vi "Image_from_name.vi"(8 "error in (no error)":errorcluster, 10 "Chemical Name":string) -> (0 "error out":errorcluster, 1 "24-bit pixmap":u32[][](array[numeric]) format="%x", 2 "Downloaded Picture":picture)   [LabVIEW 2015]
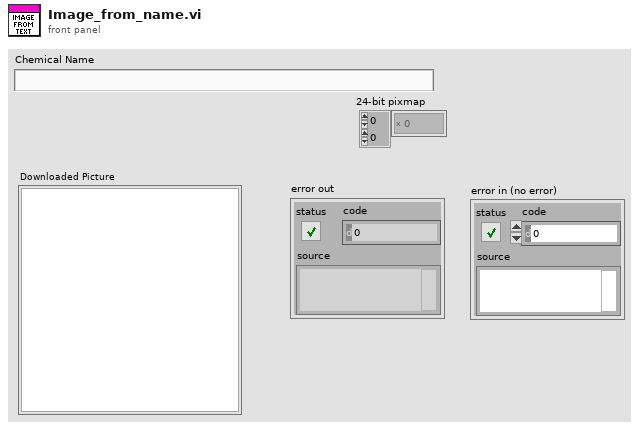
[diagram p1: front panel]
types:
  T1 = enum16{"open", "open or create", "create or replace", "create", "open (read only)"}
  T2 = typedef "imagedata.ctl" = cluster{"image type":i32, "image depth":i32, "image":u8[], "mask":u8[], "colors":u32[], "Rectangle":cluster{"left":i16, "top":i16, "right":i16, "bottom":i16}}
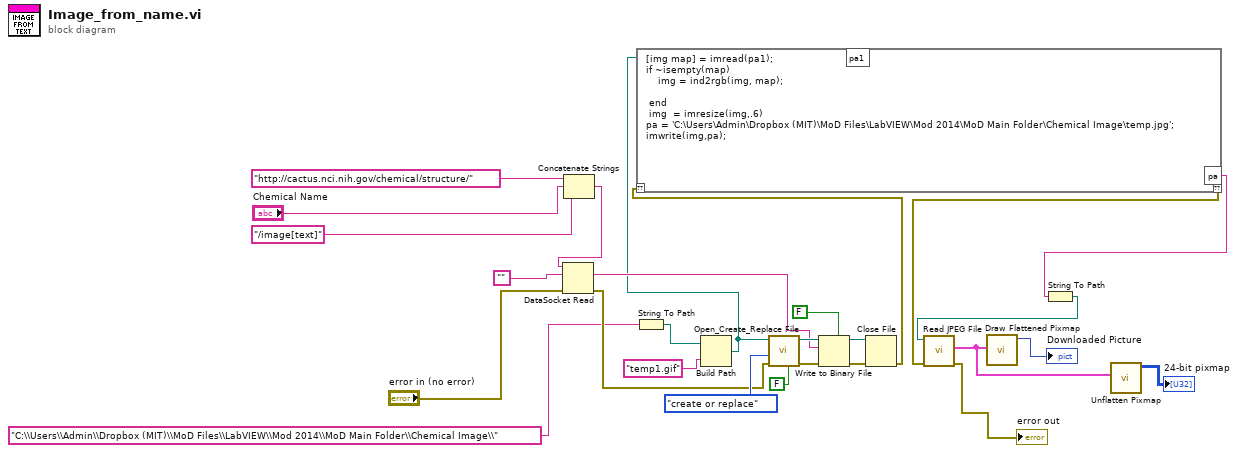
[diagram p0: block diagram]
diagram:
  n1 = Concatenate Strings("http://cactus.nci.nih.gov/chemical/structure/", "Chemical Name", "/image[text]") -> (w5:string)
  n2 = DataSocket Read(8:"error in (no error)", 10:"", 11:w5) -> (0:w18:errorcluster, 2:w14:string)  [unwired: 2 in, 5 out]
  n3 = String To Path(string="C:\\Users\\Admin\\Dropbox (MIT)\\MoD Files\\LabVIEW\\Mod 2014\\MoD Main Folder\\Chemical Image\\") -> (path=w1:path)
  n4 = Build Path(base path=w1, name or relative path="temp1.gif") -> (appended path=w9:path)
  n5 = call <vilib>:"Open_Create_Replace File.vi"("advisory dialog? (display:T)"=FALSE, "error in (no error)"=w18, "function (open:0)"=T1."create or replace", "file path"=w9) -> ("error out"=w24:errorcluster, "refnum"=w25:refnum<file>)  [unwired: 3 in, 3 out]
  n6 = Write to Binary File(file (use dialog)=w25, data=w14, error in=w24, 5:FALSE ("prepend array or string size? (T)")) -> (refnum out=w21:refnum<file>, error out=w20:errorcluster)  [unwired: 3 out]
  n7 = Close File(refnum=w21, error in=w20) -> (error out=w12:errorcluster)  [unwired: 1 out]
  n8 = script code="[img map] = imread(pa1);\nif ~isempty(map)\n    img = ind2rgb(img, map);\n   \n end\n img  = imresize(img,.6)\npa = 'C:\\Users\\Admin\\Dropbox (MIT)\\MoD Files\\LabVIEW\\Mod 2014\\MoD Main Folder\\Chemical Image\\temp.jpg';\nimwrite(img,pa);"("??"=w12, "pa1"=w9) -> ("??"=w11:errorcluster, "pa"=w13:string)
  n9 = String To Path(string=w13) -> (path=w10:path)
  n10 = call <vilib>:"Read JPEG File.vi"("error in (no error)"=w11, "path to JPEG file"=w10) -> ("error out"=→"error out":errorcluster, "image data"=w3:T2)  [unwired: 8 out]
  n11 = call <vilib>:"Draw Flattened Pixmap.vi"("image data"=w3) -> ("new picture"=→"Downloaded Picture":picture)  [unwired: 3 in, 5 out]
  n12 = call <vilib>:"Unflatten Pixmap.vi"("image data"=w3) -> ("24-bit pixmap"=→"24-bit pixmap":u32[][])  [unwired: 4 in, 6 out]
